vi "Call Root.vi"(4 "UID":string, 9 "Msg Self":refnum<class "Msg Self.lvclass">, 10 "Root Actors":refnum<class "Root Actors.lvclass">) -> (0 "Error out":errorcluster, 5 "Actor out":refnum<class "Actor.lvclass">)   [LabVIEW 2020, in "jettl.lvlib" / "Spawn.lvlib"]
uses:
  Actor/Actor.lvclass
  Msg Self/Msg Self.lvclass
  Root Actors/Root Actors.lvclass
  Attributes Metadata/Attributes Metadata.lvclass
  Async Elements/Async Elements.lvclass
  Transport/Transport.lvclass
  Attributes/Attributes.lvclass
  Msg/Msg.lvclass
  Spawn/Spawn.lvlib
  Base Attributes/Base Attributes.lvlib
  Msgs.ctl
  jettl.lvlib
  Attributes.ctl
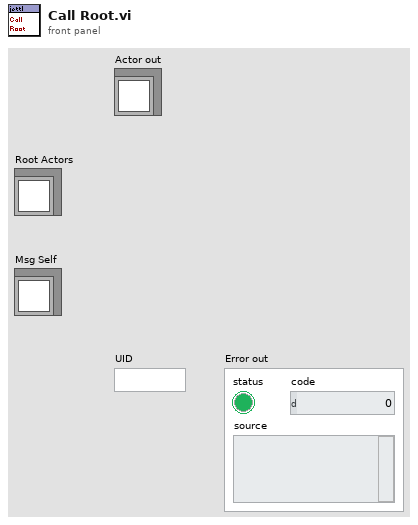
[diagram p1: front panel]
types:
  T1 = typedef "jettl.lvlib/Attributes.ctl" = cluster{"Attributes Metadata":refnum<class "Attributes Metadata.lvclass">, "Unified Msgs":T2, "Edge Actors":refnum<class "Actor.lvclass">[], "Core Actors":refnum<class "Actor.lvclass">[], "Parent Attributes":refnum<class "Attributes.lvclass">, "Root":bool, "UID":string, "Transport":refnum<class "Transport.lvclass">, "VI Ref":refnum<vi>, "Actors":refnum<class "Actor.lvclass">[]}
  T2 = typedef "jettl.lvlib/Msgs.ctl" = set{refnum<class "Msg.lvclass">}
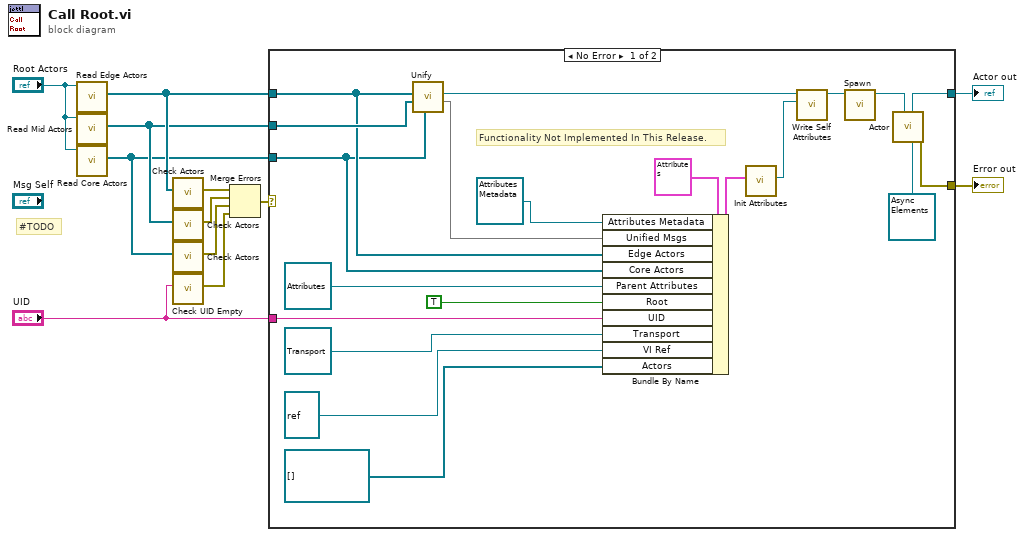
[diagram p0: block diagram]
diagram:
  # "#TODO"
  n1 = call-dynamic "Read Edge Actors.vi"("Root Actors in"="Root Actors") -> ("Edge Actors"=w4:refnum<class "Actor.lvclass">[])  [unwired: 10 in]
  n2 = call-dynamic "Read Mid Actors.vi"("Root Actors in"="Root Actors") -> ("Mid Actors"=w3:refnum<class "Actor.lvclass">[])  [unwired: 10 in]
  n3 = call-dynamic "Read Core Actors.vi"("Root Actors in"="Root Actors") -> ("Core Actors"=w2:refnum<class "Actor.lvclass">[])  [unwired: 10 in]
  n4 = call "Check Actors.vi"("Actors"=w4) -> ("Error"=w7:errorcluster)  [unwired: 10 in]
  n5 = call "Check Actors.vi"("Actors"=w3) -> ("Error"=w9:errorcluster)  [unwired: 10 in]
  n6 = call "Check Actors.vi"("Actors"=w2) -> ("Error"=w5:errorcluster)  [unwired: 10 in]
  n7 = call "Check UID Empty.vi"("UID"="UID") -> ("Error"=w8:errorcluster)  [unwired: 10 in]
  n8 = Merge Errors(w7, w9, w5, w8) -> (w10:errorcluster)
  n9 = case shown="No Error" w10 {
    selector: w10 -> [_ w33]
    tunnel: [w20 _] -> w12
    tunnel: [w21 w33] -> w11
    tunnel: w4 -> [w17 _]
    tunnel: "UID" -> [w27 _]
    tunnel: w3 -> [w18 _]
    tunnel: w2 -> [w16 _]
    frame No Error {
      # "Functionality Not Implemented In This Release."
      n10 = call "Unify.vi"("Core Actors"=w16, "Mid Actors"=w18, "Edge Actors"=w17) -> ("Unified Msgs"=w14:T2, "Unified Actor"=w15:refnum<class "Actor.lvclass">)  [unwired: 7 in]
      n11 = Bundle By Name(cluster=T1 {"Attributes Metadata"=refnum, "Unified Msgs"={}, "Edge Actors"=[], "Core Actors"=[], "Parent Attributes"=refnum, "Root"=FALSE, "UID"="", "Transport"=refnum, "VI Ref"=refnum, "Actors"=[]} ("Attributes"), "Attributes Metadata"=refnum<class "Attributes Metadata.lvclass"> refnum, "Unified Msgs"=w14, "Edge Actors"=w17, "Core Actors"=w16, "Parent Attributes"=refnum<class "Attributes.lvclass"> refnum, "Root"=TRUE, "UID"=w27, "Transport"=refnum<class "Transport.lvclass"> refnum, "VI Ref"=refnum<vi> refnum ("Actor Ref"), "Actors"=refnum<class "Actor.lvclass">[] []) -> (w24:T1)
      n12 = call "Init Attributes.vi"("Attributes"=w24) -> ("Attributes"=w32:refnum<class "Attributes.lvclass">)  [unwired: 10 in]
      n13 = call-dynamic "Write Self Attributes.vi"("Self Attributes"=w32, "Actor in"=w15) -> ("Actor out"=w23:refnum<class "Actor.lvclass">)  [unwired: 9 in]
      n14 = call-dynamic "Spawn.vi"("Actor in"=w23) -> ("Actor out"=w19:refnum<class "Actor.lvclass">)  [unwired: 10 in]
      n15 = call "Actor.vi"("Async Elements"=refnum<class "Async Elements.lvclass"> refnum, "Actor in"=w19) -> ("Error out"=w21:errorcluster, "Actor out"=w20:refnum<class "Actor.lvclass">)  [unwired: 8 in]
    }
    frame Error {
    }
  }
  "Error out" <- w11
  "Actor out" <- w12
